vi "InitVarTree.vi"(1 "dims":cluster{"name":string, "size":u64}[](array[cluster]), 2 "vars":T2(array[cluster])) -> (0 "var tree":T1(array[cluster]))   [LabVIEW 2016]
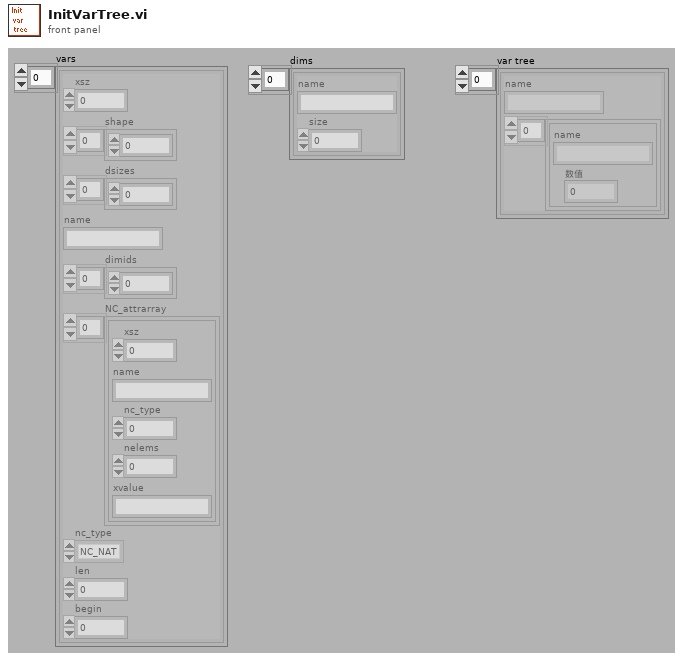
[diagram p1: front panel]
types:
  T1 = cluster{"name":string, cluster{"name":string, "数值":u64}[]}[]
  T2 = cluster{"xsz":u64, "shape":u64[], "dsizes":u64[], "name":string, "dimids":u64[], "NC_attrarray":cluster{"xsz":u64, "name":string, "nc_type":u16, "nelems":u64, "xvalue":string}[], "nc_type":enum16{"NC_NAT", "NC_BYTE", "NC_CHAR", "NC_SHORT", "NC_INT", "NC_FLOAT", "NC_DOUBLE"}, "len":u64, "begin":u64}[]
  T3 = cluster{"name":string, cluster{"name":string, "数值":u64}[]}
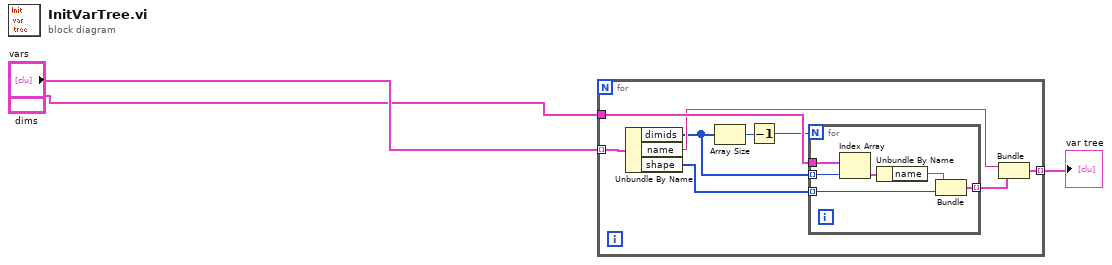
[diagram p0: block diagram]
diagram:
  n1 = for {
    tunnel: "vars" -> [w12] mode=indexing
    tunnel: "dims" -> [w11]
    tunnel: [w4] -> w1 mode=indexing
    n2 = Unbundle By Name(w12) -> ("dimids"=w8:u64[], "name"=w10:string, "shape"=w6:u64[])
    n3 = Array Size(array=w8) -> (size(s)=w9:i32)
    n4 = Decrement(x=w9) -> (x-1=w7:i32)
    n5 = for {
      N: w7 -> [_]
      tunnel: w8 -> [w17] mode=indexing
      tunnel: w11 -> [w18]
      tunnel: w6 -> [w14] mode=indexing
      tunnel: [w13] -> w5 mode=indexing
      n6 = Index Array(array=w18, index=w17) -> (element=w16:cluster{"name":string, "size":u64})
      n7 = Unbundle By Name(w16) -> ("name"=w15:string)
      n8 = Bundle("name"=w15, "数值"=w14) -> (w13:cluster{"name":string, "数值":u64})  [unwired: 1 out]
    }
    n9 = Bundle("name"=w10, w5) -> (w4:T3)  [unwired: 1 out]
  }
  "var tree" <- w1
